vi "Set Background id.vi"(8 "error in":errorcluster, 10 "id":string, 11 "Inset in":refnum<class "Inset.lvclass">) -> (0 "error out":errorcluster, 3 "Inset out":refnum<class "Inset.lvclass">)   [LabVIEW 2019, in "Inset.lvclass"]
uses:
  Inset.lvclass
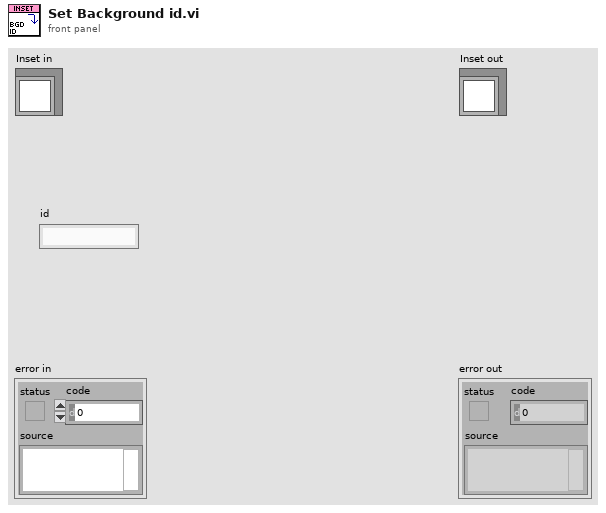
[diagram p1: front panel]
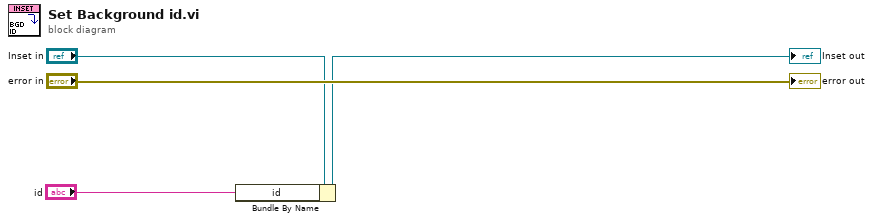
[diagram p0: block diagram]
diagram:
  n1 = Bundle By Name(cluster="Inset in", "id"="id") -> (→"Inset out":refnum<class "Inset.lvclass">)
  "error out" <- "error in"
